vi "String to U16.vi"(8 "error in":errorcluster, 11 "String":string) -> (0 "error out":errorcluster, 3 "U16":u16)   [LabVIEW 2024, in "Electronic Datasheet.lvlib"]
doc: "A string that contains the number to convert."
uses:
  Electronic Datasheet.lvlib
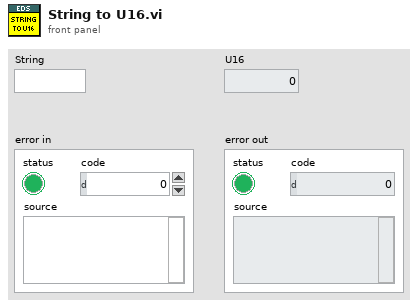
[diagram p1: front panel]
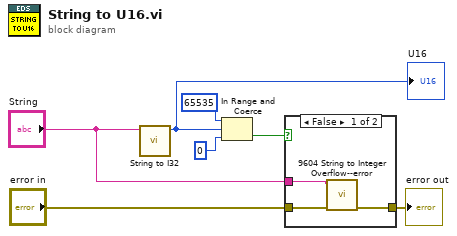
[diagram p0: block diagram]
diagram:
  n1 = call "String to I32.vi"("String"="String") -> ("I32"=w4:i32)  [unwired: 10 in]
  "U16" <- w4
  n2 = In Range and Coerce(upper limit=65535, x=w4, lower limit=0) -> (In Range?=w5:bool)  [unwired: 1 out]
  n3 = case shown="False" w5 {
    tunnel: "error in" -> [w10 w11]
    tunnel: [w9 w11] -> w2
    tunnel: "String" -> [w8 _]
    frame False {
      n4 = call "9604 String to Integer Overflow--error.vi"("error in"=w10, "Integer String"=w8) -> ("error out"=w9:errorcluster)  [unwired: 9 in]
    }
    frame True {
    }
  }
  "error out" <- w2
